vi "serial_read_and_write.vi"(0 "write buffer":string) -> (2 "unsigned byte array":u8[](array[numeric]))   [LabVIEW 2011]
uses:
  <vilib>/Instr/_visa.llb/VISA Configure Serial Port (Instr).vi
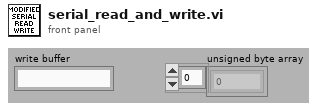
[diagram p1: front panel]
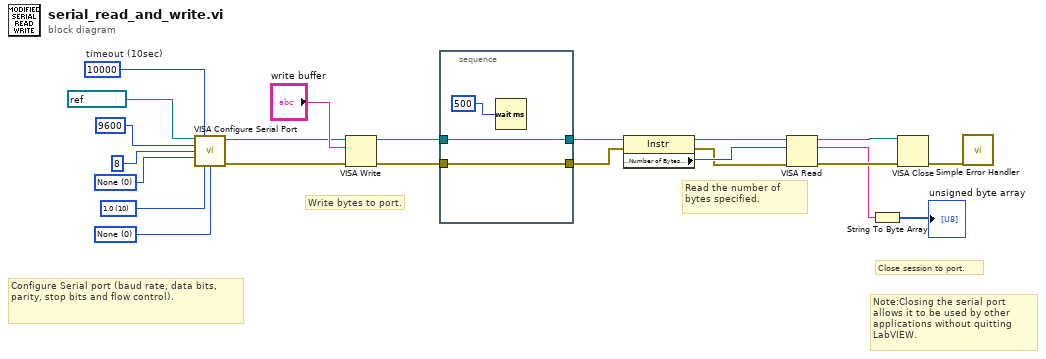
[diagram p0: block diagram]
diagram:
  w13 = u16 0 items=["None"=0, "XON/XOFF"=1, "RTS/CTS"=2, "DTR/DSR"=4] ("flow control")
  w12 = u16 10 items=["1.0"=10, "1.5"=15, "2.0"=20] ("stop bits")
  w10 = u16 0 items=["None", "Odd", "Even", "Mark", "Space"] ("parity")
  w11 = u32 10000  # timeout (10sec)
  # "Read the number of bytes specified."
  # "Write bytes to port."
  # "Note:Closing the serial port allows it to be used by other applications without quitting LabVIEW."
  # "Configure Serial port (baud rate, data bits, parity, stop bits and flow control)."
  # "Close session to port."
  n1 = call-poly "VISA Configure Serial Port"("VISA resource name"=refnum<visa-resource-name> "ASRL3", "timeout (10sec)"=w11, "baud rate (9600)"=u32 9600 ("baud rate"), "data bits (8)"=u16 8 ("data bits"), "parity (0:none)"=w10, "stop bits (10: 1 bit)"=w12, "flow control (0:none)"=w13) -> ("VISA resource name out"=w6:refnum<visa-resource-name>, "error out"=w5:errorcluster)  [unwired: 2 in, 5 out]
  n2 = VISA Write(VISA resource name=w6, write buffer="write buffer", error in (no error)=w5) -> (VISA resource name out=w17:refnum<visa-resource-name>, error out=w15:errorcluster)  [unwired: 1 out]
  n3 = stacked-sequence {
    tunnel: w15 -> [w25]
    tunnel: [w25] -> w16
    tunnel: w17 -> [w24]
    tunnel: [w24] -> w18
    frame #0 {
      n4 = Wait (ms)(milliseconds to wait=u32 500 ("delay before read (ms)")) -> ()  [unwired: 1 out]
    }
  }
  n5 = property class="Instr"(reference=w18, error in=w16) -> (reference out=w20:refnum<visa-resource-name>, error out=w21:errorcluster, "Serial Settings:Number of Bytes at Serial Port"=w22:u32)
  n6 = VISA Read(VISA resource name=w20, byte count=w22, error in (no error)=w21) -> (VISA resource name out=w8:refnum<visa-resource-name>, read buffer=w1:string, error out=w7:errorcluster)  [unwired: 1 out]
  n7 = String To Byte Array(string=w1) -> (unsigned byte array=→"unsigned byte array":u8[])
  n8 = VISA Close(VISA resource name=w8, error in (no error)=w7) -> (error out=w9:errorcluster)
  n9 = call <vilib>:"Simple Error Handler.vi"("error in (no error)"=w9) -> ()  [unwired: 1 in, 8 out]
